vi "Move Robot on Grid.vi"(5 "Density Check":i32=4, 7 "New Pos":T1, 10 "Currnt Pos":T1, 11 "Array in":i32[][](array[numeric])) -> (2 "Density Check Met":bool, 3 "Array out":i32[][](array[numeric]))   [LabVIEW 2024]
uses:
  Utility/Universal Utility/TypeDefs_Utility/Cluster_Row-Column.ctl
  Utility/Universal Utility/TypeDefs_Utility/ENUM_8 Directions U-D-L-R.ctl
  8d28afed-0a2f-4dcf-bf59-0e85d1ed97ce.vi
  <vilib>/Utility/error.llb/Trim Whitespace.vi
  <vilib>/Utility/error.llb/Trim Whitespace One-Sided.vi
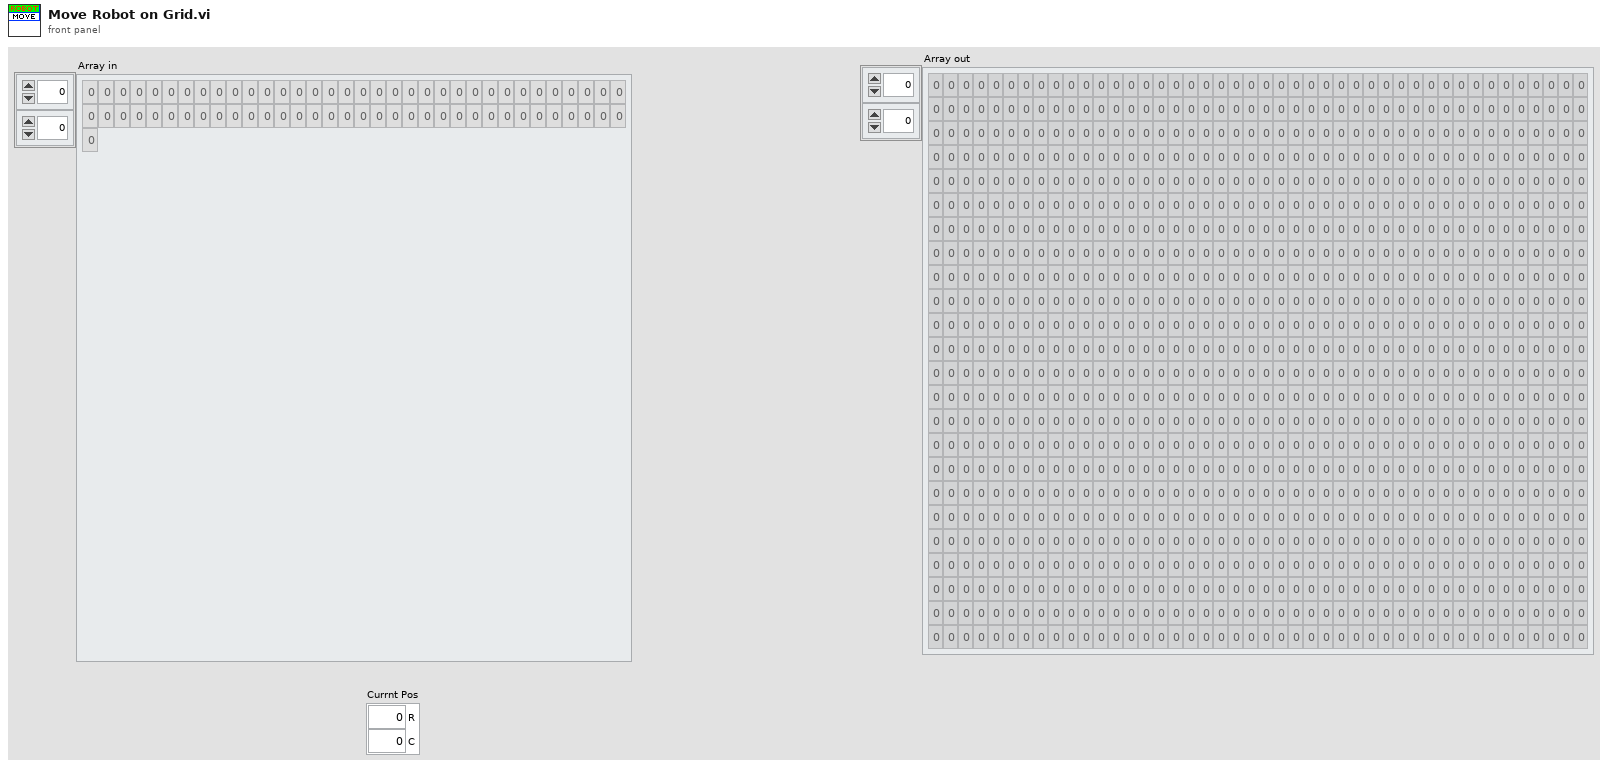
[diagram p1: front panel]
types:
  T1 = typedef "Cluster_Row-Column.ctl" = cluster{"R":i32, "C":i32}
  T2 = typedef "ENUM_8 Directions U-D-L-R.ctl" = enum16{"Up;-1,0", "Up-Right;-1,1", "Right;0,1", "Down-Right;1,1", "Down;1,0", "Down-Left;1,-1", "Left;0,-1", "Up-Left;-1,-1"}
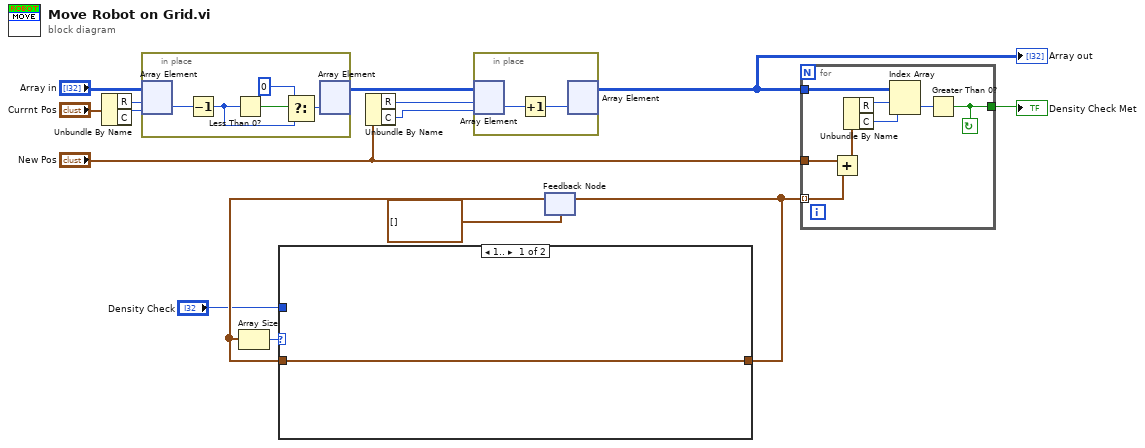
[diagram p0: block diagram]
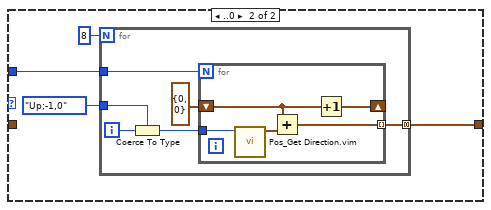
[diagram p2: hidden frame]
diagram:
  n1 = Unbundle By Name("Currnt Pos") -> ("R"=w12:i32, "C"=w13:i32)
  n2 = in-place {
    n3 = in-place-array #1("Array in", w12, w13) -> (w20:i32)
    n4 = Decrement(x=w20) -> (x-1=w18:i32)
    n5 = Less Than 0?(x=w18) -> (x < 0?=w19:bool)
    n6 = Select(t=0, s=w19, f=w18) -> (s? t:f=w16:i32)
    n7 = in-place-array #1(w16) -> (w11:i32[][])  [unwired: 2 out]
  }
  n8 = Unbundle By Name("New Pos") -> ("R"=w10:i32, "C"=w9:i32)
  n9 = in-place {
    n10 = in-place-array #2(w11, w10, w9) -> (w22:i32)
    n11 = Increment(x=w22) -> (x+1=w21:i32)
    n12 = in-place-array #2(w21) -> (w4:i32[][])  [unwired: 2 out]
  }
  "Array out" <- w4
  n13 = feedback #3(T1[] []) -> (w7:T1[])
  n14 = Array Size(array=w7) -> (size(s)=w6:i32)
  n15 = case shown="1.." w6 {
    tunnel: w7 -> [w23 _]
    tunnel: [w23 w25] -> w3
    tunnel: "Density Check" -> [_ w24]
    frame 1.. {
    }
    frame ..0 {
      n16 = for {
        N: 8 -> [_]
        tunnel: ENUM_8_Directions_U-D-L-R."Up;-1,0" ("Direction 8") -> [w32]
        tunnel: [w29] -> w25 mode=concatenating
        tunnel: w24 -> [w28]
        i -> [w33]
        n17 = Coerce To Type(0:w33, 1:w32) -> (2:w31:T2)
        n18 = for {
          N: w28 -> [_]
          tunnel: w31 -> [w38]
          shift-right: [w34] -> _
          shift-left: T1 {"R"=0, "C"=0} ("Position") -> [w35]
          tunnel: [w36] -> w29 mode=indexing
          n19 = call "Pos_Get Direction.vim"("Direction"=w38) -> ("Position"=w37:T1)  [unwired: 10 in]
          n20 = Add(x=w35, y=w37) -> (x+y=w36:T1)
          n21 = Increment(x=w35) -> (x+1=w34:T1)
        }
      }
    }
  }
  n22 = feedback-in #3(w3) -> ()
  n23 = for {
    tunnel: "New Pos" -> [w46]
    tunnel: w4 -> [w43]
    tunnel: w3 -> [w45] mode=indexing
    tunnel: [w39] -> w2
    stop <- w39 continue-if-true
    n24 = Add(x=w46, y=w45) -> (x+y=w44:T1)
    n25 = Unbundle By Name(w44) -> ("R"=w42:i32, "C"=w41:i32)
    n26 = Index Array(array=w43, index (row)=w42, index (col)=w41) -> (element=w40:i32)
    n27 = Greater Than 0?(x=w40) -> (x > 0?=w39:bool)
  }
  "Density Check Met" <- w2
